vi "Get System Name.vi"(8 "error in (no error)":errorcluster, 11 "Pressure in":refnum<class "Pressure.lvclass">) -> (0 "error out":errorcluster, 2 "System Name":string, 3 "Pressure out":refnum<class "Pressure.lvclass">)   [LabVIEW 2014, in "Pressure.lvlib" / "Pressure.lvclass"]
uses:
  Pressure.lvclass
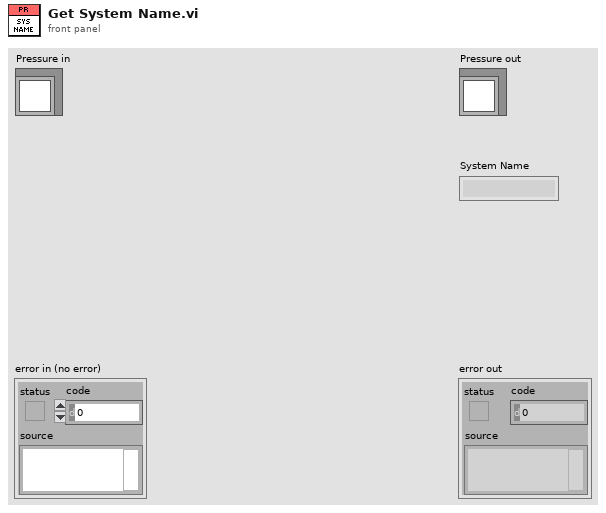
[diagram p1: front panel]
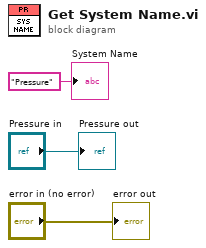
[diagram p0: block diagram]
diagram:
  "error out" <- "error in (no error)"
  "Pressure out" <- "Pressure in"
  "System Name" <- "Pressure"
